vi "sub_SDR_mimo_DemuxPorts.vi"(10 "Data in (2D)":cdb[][](array[numeric])) -> (0 "Port 2":cdb[](array[numeric]), 3 "Port 1":cdb[](array[numeric]))   [LabVIEW 2012]
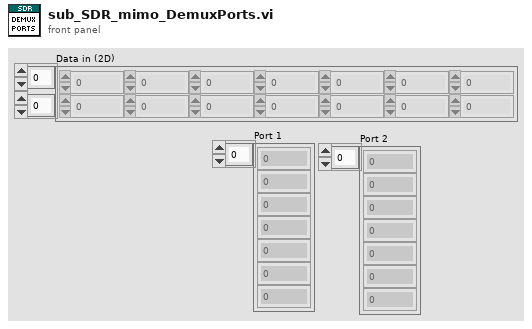
[diagram p1: front panel]
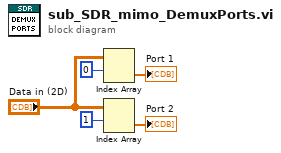
[diagram p0: block diagram]
diagram:
  n1 = Index Array(array="Data in (2D)", index (row)=0 ("index")) -> (element=→"Port 1":cdb[])  [unwired: 1 in]
  n2 = Index Array(array="Data in (2D)", index (row)=1 ("index")) -> (element=→"Port 2":cdb[])  [unwired: 1 in]
